vi "Read Product Family.vi"(8 "error in (no error)":errorcluster, 11 "Lutron QS Object in":refnum<class "Lutron QS Object.lvclass">) -> (0 "error out":errorcluster, 2 "Product Family":string, 3 "Lutron QS Object out":refnum<class "Lutron QS Object.lvclass">)   [LabVIEW 2016, in "Lutron QS Control Protocol.lvlib" / "Lutron QS Object.lvclass"]
uses:
  Lutron QS Object.lvclass
  Lutron QS Object.lvclass/Lutron QS Object.ctl
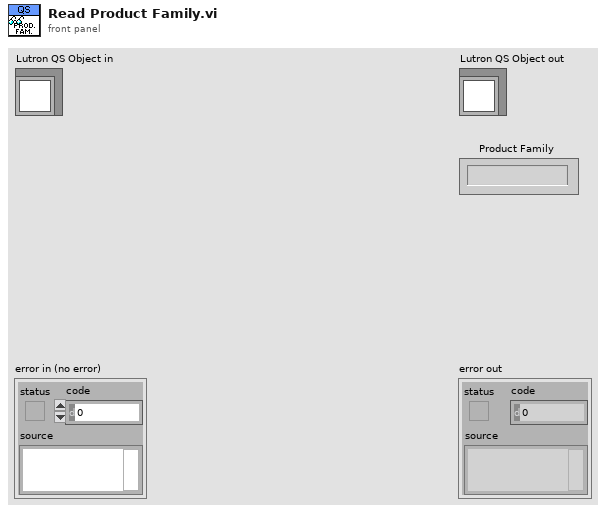
[diagram p1: front panel]
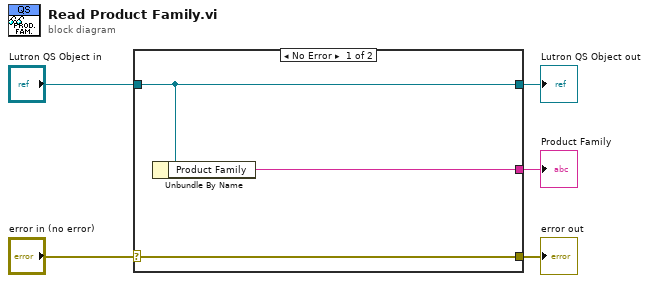
[diagram p0: block diagram]
diagram:
  n1 = case shown="No Error" "error in (no error)" {
    selector: "error in (no error)" -> [w8 w9]
    tunnel: [w8 w9] -> w4
    tunnel: [w7 w10] -> w2
    tunnel: "Lutron QS Object in" -> [w7 w10]
    tunnel: [w6 _] -> w1
    frame No Error {
      n2 = Unbundle By Name(w7) -> ("Product Family"=w6:string)
    }
    frame Error {
    }
  }
  "error out" <- w4
  "Lutron QS Object out" <- w2
  "Product Family" <- w1
